vi "Delete Empty Case Structure Frames.vi"(8 "error in (no error)":errorcluster, 11 "CaseStructure in":refnum<vi>) -> (0 "error out":errorcluster, 3 "CaseStructure out":refnum<vi>)   [LabVIEW 2019, in "gRPC Template Creation Utility.lvlib"]
uses:
  gRPC Template Creation Utility.lvlib
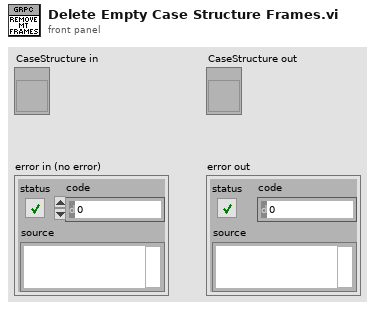
[diagram p1: front panel]
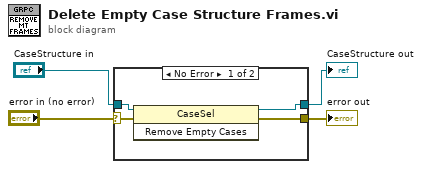
[diagram p0: block diagram]
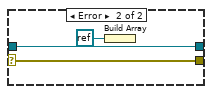
[diagram p2: hidden frame]
diagram:
  n1 = case shown="No Error" "error in (no error)" {
    selector: "error in (no error)" -> [w6 w11]
    tunnel: [w7 w9] -> w4
    tunnel: [w5 w11] -> w3
    tunnel: "CaseStructure in" -> [w8 w9]
    frame No Error {
      n2 = invoke class="CaseSel" method="Remove Empty Cases"(reference=w8, error in=w6) -> (reference out=w7:refnum<vi>, error out=w5:errorcluster)  [unwired: 1 in, 1 out]
    }
    frame Error {
      n3 = Build Array(refnum<k0> refnum) -> ()  [unwired: 1 out]
    }
  }
  "error out" <- w3
  "CaseStructure out" <- w4
